vi "DigitalDemultiplexerV3.vi"() -> ()   [LabVIEW 2012]
uses:
  <vilib>/Platform/TimedLoop/XDataNode/timing_clust.ctl
  <vilib>/Platform/TimedLoop/XDataNode/nitl_modes.ctl
  <vilib>/Platform/TimedLoop/XDataNode/wakeup.ctl
  <vilib>/rvi/Emulation/niFpgaSctlEmulationRegisterWithScheduler.vi
  <vilib>/rvi/eio/common/nirviEmuTemplateMethod_errors.vi
  <vilib>/rvi/Emulation/niFpgaSctlEmulationScheduler.vi
  <vilib>/rvi/FIFO/Fifo_Resource/nirvififoEmulationSetSize.vi
  <vilib>/rvi/DataTransferAndStorage/Container/Common/niFpgaContainerGetUniqueNameForEmu.vi
  <vilib>/rvi/errors/niFpgaSetErrorForExecOnDevCompSimple.vi
  <vilib>/rvi/eio/common/nirviEmuReportErrorAndStop.vi
  <vilib>/rvi/Emulation/niFpgaSctlEmulationFifoFullMgr.vi
  <vilib>/rvi/Emulation/niFpgaSctlEmulationResourceMgr.vi
  <vilib>/rvi/interface/RandomDataEmulation/nirviRandomDataFPGAFIFO.vi
  <vilib>/rvi/interface/RandomDataEmulation/niFpgaRandomDataHandleErrors.vi
  <vilib>/rvi/Emulation/niFpgaSctlEmulationGlobalWrite.vi
  <vilib>/Platform/TimedLoop/XDataNode/XDataNode.xnode
  <vilib>/eio/EIONode/EIONode.xnode
  <vilib>/rvi/DataTransferAndStorage/Container/XNode/niFpgaContainer.xnode
  <vilib>/rvi/FIFO/Fifo_Resource/nirvififoEmulationClear.vi
  <vilib>/rvi/FIFO/Fifo_Resource/nirvififoEmulationWrite.vi
  <vilib>/rvi/FIFO/Fifo_Resource/nirvififoEmulationRead.vi
  <vilib>/rvi/interface/RandomDataEmulation/nirviRandomDataFpgaReadWriteTemplate.vi
  <vilib>/Platform/TimedLoop/XDataNode/XDNodeRunTimeDep.lvlib
panel:
  in  "Count mode":bool
  out "Laser pulses per pixel A1":u16
  out "ToHost FIFO Overflow A2Ch2":bool
  out "ToHost FIFO Overflow A2Ch1":bool
  out "ToHost FIFO Overflow A1Ch2":bool
  in  "Samples per pixel Acq A2":u16=10000 caption="Samples per pixel Acq"
  in  "Samples per pixel Acq A1":u16=10000 caption="Samples per pixel Acq"
  in  "Requested pixels A2":u32=100000 caption="Requested pixels"
  in  "Samples per pixel A2":u16=10000 caption="Samples per pixel"
  out "ToHost FIFO Overflow A1Ch1":bool
  out "Acquiring":bool
  in  "Wait for trigger":bool
  in  "Acquire continuously":bool=TRUE
  in  "Requested pixels A1":u32=100000 caption="Requested pixels"
  in  "Clear Interloop FIFO":bool
  out "Interloop FIFO overflow":bool
  in  "Samples per pixel A1":u16=10000 caption="Samples per pixel"
  in  "Acquire":bool
  out "Interloop FIFO timeout":bool
  in  "Commit":bool
  out "Xpoint_Switch_Ready":bool
  in  "Xpoint_Switch_Write":bool
  in  "Clock Source":u8(ring)=3 items=["Tristate"=0, "Sync Clock (PXIe only)"=2, "Adapter Module Onboard Clock"=3, "Strobe from Crosspoint Switch"=4, "Strobe Bypass"=5]
  in  "Onboard_Clock_Write":bool
  in  "Onboard_Clock_Write_Data":u16
  out "Onboard_Clock_Ready":bool
  in  "Acq_Reset":bool
  # "6587 IO module configuration"
  # "Digital Demultiplexer V3 - very simple 160, count high or flanks"
  # "Acquisition control"
  # "Area 1"
  # "Area 2"
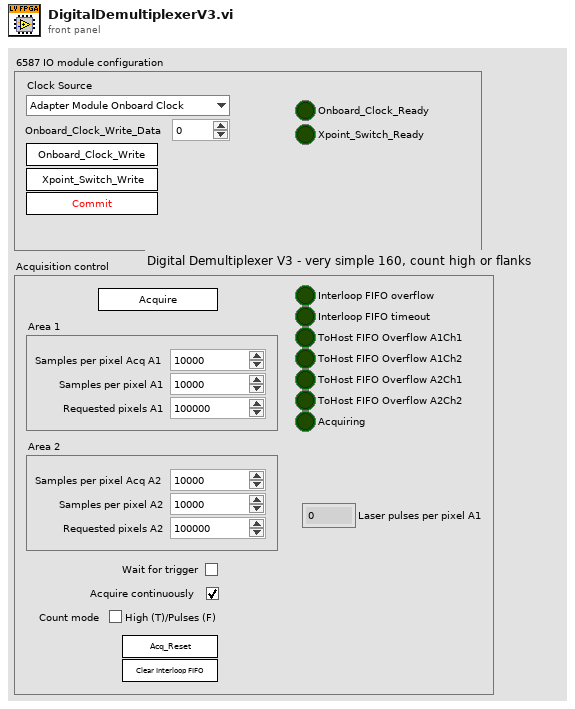
[diagram p1: front panel]
types:
  T1 = typedef "XDNodeRunTimeDep.lvlib/timing_clust.ctl" = cluster{"Expected End [f-1]":u64, "Actual End [f-1]":u64, "Finished Late? [f-1]":bool, "Expected End [i-1]":u64, "Actual End [i-1]":u64, "Finished Late? [i-1]":bool, "Expected Start [i]":u64, "Actual Start [i]":u64, "Expected Start [f]":u64, "Actual Start [f]":u64, "Source Name":string, "Structure Name":string, "Period":i64, "Deadline":i64, "Offset":i64, "Start":i64, "Priority":i32, "Timeout":i32, "Mode":T2, "Wakeup Reason":T3, "Error":errorcluster, "Source Type":string, "Secondary Source Type":string, "Global End Time":u64, "Global Start Time":u64, "Frame Duration":u64, "Iteration Duration":u64, "Assigned CPU":i32, "I/O Scan Engine Mode":u32}
  T2 = typedef "XDNodeRunTimeDep.lvlib/nitl_modes.ctl" = enum32{"No Change", "Process missed periods, maintain original phase", "Discard missed periods, maintain original phase", "Process missed periods, ignore original phase", "Discard missed periods, ignore original phase"}
  T3 = typedef "XDNodeRunTimeDep.lvlib/wakeup.ctl" = enum32{"Normal", "Aborted", "Asynchronous wakeup", "Timing source error", "Timed loop error", "Timeout"}
  T4 = cluster{"Laser":u64, "A1Ch1":u64, "A1Ch2":u64, "A2Ch1":u64, "A2Ch2":u64}
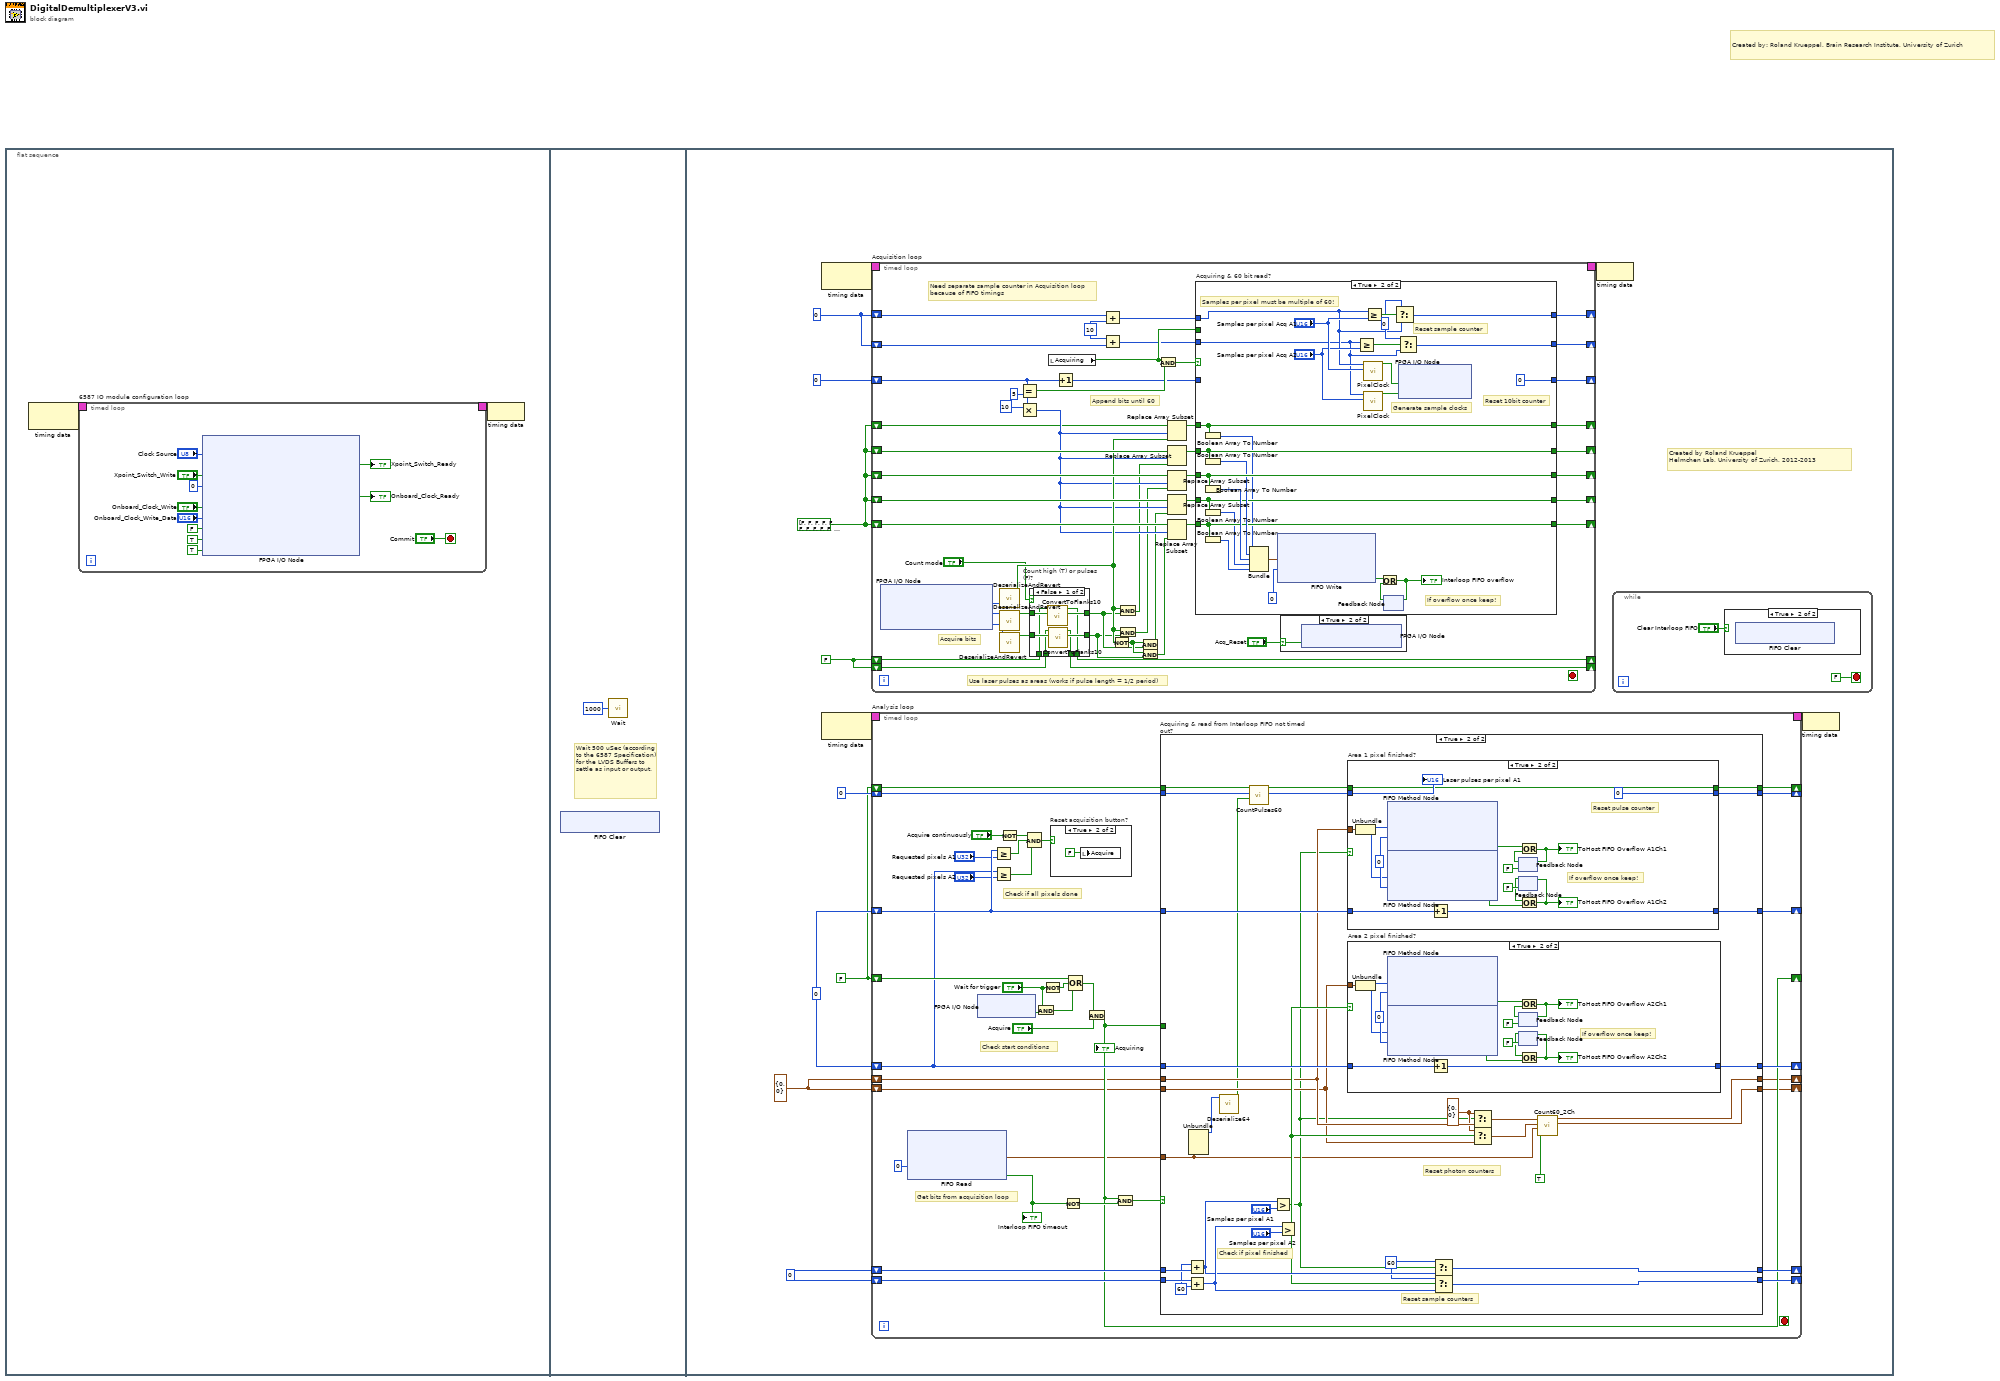
[diagram p0: block diagram]
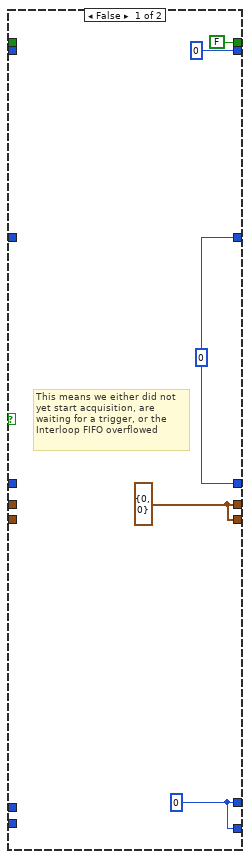
[diagram p5: hidden frame]
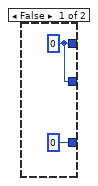
[diagram p11: hidden frame]
diagram:
  # "Created by: Roland Krueppel, Brain Research Institute, University of Zurich"
  n1 = flat-sequence {
    frame #0 {
      n2 = node-c288() -> (w2:T1)  [unwired: 1 in]
      n3 = timed-loop "6587 IO module configuration loop" {
        timing: w2 -> [_]
        timing-out: [_] -> w1
        stop <- "Commit" stop-if-true
        n4 = xnode "FPGA I/O Node"("IO Module\\Acq_IO_Clock_Source"="Clock Source", "IO Module\\Xpoint_Switch_Write"="Xpoint_Switch_Write", "IO Module\\LVDS_Data_Dir"=u16 0 ("IO Module\\LVDS_Data_Dir"), "IO Module\\Onboard_Clock_Write"="Onboard_Clock_Write", "IO Module\\Onboard_Clock_Write_Data"="Onboard_Clock_Write_Data", "IO Module\\SE_PFI0_WE"=FALSE ("IO Module\\SE_PFI0_WE"), "IO Module\\SE_PFI1_WE"=TRUE ("IO Module\\SE_PFI1_WE"), "IO Module\\SE_PFI2_WE"=TRUE ("IO Module\\SE_PFI2_WE")) -> ("IO Module\\Xpoint_Switch_Ready"=→"Xpoint_Switch_Ready":bool, "IO Module\\Onboard_Clock_Ready"=→"Onboard_Clock_Ready":bool)  [unwired: 10 in, 10 out]
      }
      n5 = node-c288(w1) -> ()
    }
    frame #1 {
      # "Wait 500 uSec (according to the 6587 Specification) for the LVDS Buffers to settle as input or output."
      n6 = xnode ("FIFO Clear")() -> ()  [unwired: 1 in, 1 out]
      n7 = call "Wait"("Count(uSec)"=u32 1000) -> ()  [unwired: 1 out]
    }
    frame #2 {
      w19 = FALSE
      w24 = cluster{u16, u16} {0, 0} ("output cluster")
      w25 = u16 0
      w23 = u32 0 ("Cycle counter out")
      w26 = u16 0
      w22 = bool[] [FALSE, FALSE, FALSE, FALSE, FALSE, FALSE, FALSE, FALSE, FALSE, FALSE, FALSE, FALSE, FALSE, FALSE, FALSE, FALSE, FALSE, FALSE, FALSE, FALSE, FALSE, FALSE, FALSE, FALSE, FALSE, FALSE, FALSE, FALSE, FALSE, FALSE, FALSE, FALSE, FALSE, FALSE, FALSE, FALSE, FALSE, FALSE, FALSE, FALSE, FALSE, FALSE, FALSE, FALSE, FALSE, FALSE, FALSE, FALSE, FALSE, FALSE, FALSE, FALSE, FALSE, FALSE, FALSE, FALSE, FALSE, FALSE, FALSE, FALSE, FALSE, FALSE, FALSE, FALSE] ("Boolean array")
      w20 = FALSE ("Last laser bit out")
      # "Created by Roland Krueppel\nHelmchen Lab, University of Zurich, 2012-2013"
      n8 = node-c288() -> (w31:T1)  [unwired: 1 in]
      n9 = node-c288() -> (w29:T1)  [unwired: 1 in]
      n10 = timed-loop "Acquisition loop" {
        timing: w31 -> [_]
        timing-out: [_] -> w30
        shift-right: [w216] -> _
        shift-left: w22 -> [w222]
        shift-right: [w215] -> _
        shift-left: 0 -> [w214]
        shift-right: [w211] -> _
        shift-left: w22 -> [w213]
        shift-right: [w210] -> _
        shift-left: w25 -> [w203]
        shift-right: [w209] -> _
        shift-left: w25 -> [w201]
        shift-right: [w192] -> _
        shift-left: w22 -> [w197]
        shift-right: [w191] -> _
        shift-left: w22 -> [w196]
        shift-right: [w186] -> _
        shift-left: w22 -> [w188]
        shift-right: [w175] -> _
        shift-left: w19 -> [w177]
        shift-right: [w174] -> _
        shift-left: w19 -> [w176]
        stop <- _ stop-if-true
        w199 = u16 10 ("y")
        # "Use laser pulses as areas (works if pulse length = 1/2 period)"
        # "Need separate sample counter in Acquisition loop\nbecause of FIFO timings"
        # "Append bits until 60"
        # "Acquire bits"
        n11 = xnode "FPGA I/O Node"() -> ("IO Module\\LVDS_Ch0_Rd"=w206:u16, "IO Module\\LVDS_Ch1_Rd"=w205:u16, "IO Module\\LVDS_Ch2_Rd"=w204:u16)  [unwired: 3 in, 3 out]
        n12 = call "DeserializeAndRevert.vi"("U16 input"=w206) -> ("10bit output"=w190:bool[])  [unwired: 10 in]
        n13 = call "DeserializeAndRevert.vi"("U16 input"=w205) -> ("10bit output"=w181:bool[])  [unwired: 10 in]
        n14 = call "DeserializeAndRevert.vi"("U16 input"=w204) -> ("10bit output"=w180:bool[])  [unwired: 10 in]
        n15 = Equal?(x=w214, y=5) -> (x = y?=w219:bool)
        n16 = Multiply(x=10 ("y"), y=w214) -> (x*y=w189:i32)
        n17 = case "Count high (T) or pulses (F)?" shown="False" "Count mode" {
          tunnel: w181 -> [w230 w234]
          tunnel: w180 -> [w228 w233]
          tunnel: [w229 w234] -> w179
          tunnel: [w227 w233] -> w178
          tunnel: w177 -> [w226 w231]
          tunnel: w176 -> [w225 w232]
          tunnel: [w224 w232] -> w174
          tunnel: [w223 w231] -> w175
          frame False {
            n18 = call "ConvertToFlanks10.vi"("10bit input"=w230, "Last sample in"=w226) -> ("Flank output"=w229:bool[], "Last sample out"=w223:bool)  [unwired: 8 in]
            n19 = call "ConvertToFlanks10.vi"("10bit input"=w228, "Last sample in"=w225) -> ("Flank output"=w227:bool[], "Last sample out"=w224:bool)  [unwired: 8 in]
          }
          frame True {
          }
        }
        n20 = local read "Acquiring"() -> (w208:bool)
        n21 = Increment(x=w214) -> (x+1=w207:i32)
        n22 = Add(x=w203, y=w199) -> (x+y=w202:u16)
        n23 = Add(x=w199, y=w201) -> (x+y=w200:u16)
        n24 = Not(x=w190) -> (.not. x?=w195:bool[])
        n25 = And(x=w190, y=w179) -> (x .and. y?=w185:bool[])
        n26 = And(x=w190, y=w178) -> (x .and. y?=w184:bool[])
        n27 = And(x=w195, y=w179) -> (x .and. y?=w183:bool[])
        n28 = And(x=w195, y=w178) -> (x .and. y?=w182:bool[])
        n29 = And(x=w208, y=w219) -> (x .and. y?=w218:bool)
        n30 = Replace Array Subset(array=w188, new element=w190, index=w189) -> (w187:bool[])
        n31 = Replace Array Subset(array=w222, new element=w185, index=w189) -> (w217:bool[])
        n32 = Replace Array Subset(array=w213, new element=w184, index=w189) -> (w212:bool[])
        n33 = Replace Array Subset(array=w197, new element=w183, index=w189) -> (w194:bool[])
        n34 = Replace Array Subset(array=w196, new element=w182, index=w189) -> (w193:bool[])
        n35 = case "Acquiring & 60 bit read?" shown="True" w218 {
          tunnel: w217 -> [w247 w278]
          tunnel: [w247 w278] -> w216
          tunnel: [w239 0] -> w215
          tunnel: w207 -> [w240 _]
          tunnel: w212 -> [w246 w277]
          tunnel: [w246 w277] -> w211
          tunnel: w202 -> [w244 w266]
          tunnel: [w241 w275] -> w210
          tunnel: w200 -> [w243 w265]
          tunnel: [w242 w270] -> w209
          tunnel: w208 -> [w245 _]
          tunnel: w194 -> [w238 w259]
          tunnel: w193 -> [w237 w258]
          tunnel: [w238 w259] -> w192
          tunnel: [w237 w258] -> w191
          tunnel: w187 -> [w236 w254]
          tunnel: [w236 w254] -> w186
          frame False {
            n36 = case "Acquiring?" shown="True" w245 {
              tunnel: w244 -> [_ w252]
              tunnel: w243 -> [_ w251]
              tunnel: [w249 w252] -> w241
              tunnel: [w249 w251] -> w242
              tunnel: w240 -> [_ w250]
              tunnel: [0 w250] -> w239
              frame False {
                w249 = u16 0
              }
              frame True {
              }
            }
          }
          frame True {
            w271 = u16 0 ("t")
            # "Reset 10bit counter"
            # "Samples per pixel must be multiple of 60!"
            # "Reset sample counter"
            # "If overflow once keep!"
            # "Generate sample clocks"
            n37 = Boolean Array To Number(Boolean array=w254) -> (number=w253:u64)
            n38 = Boolean Array To Number(Boolean array=w278) -> (number=w261:u64)
            n39 = Boolean Array To Number(Boolean array=w277) -> (number=w260:u64)
            n40 = Boolean Array To Number(Boolean array=w259) -> (number=w257:u64)
            n41 = Boolean Array To Number(Boolean array=w258) -> (number=w256:u64)
            n42 = Bundle(w253, w261, w260, w257, w256) -> (w255:cluster{u64, u64, u64, u64, u64})  [unwired: 1 in]
            n43 = xnode ("FIFO Write")("Element"=w255, "Timeout"=0) -> ("Timed Out?"=w264:bool)  [unwired: 1 in, 1 out]
            n44 = Greater Or Equal?(x=w265, y="Samples per pixel Acq A2") -> (x >= y?=w272:bool)
            n45 = call "PixelClock.vi"("Samples per pixel"="Samples per pixel Acq A1", "Sample counter"=w266) -> ("Pixel clock"=w273:bool)  [unwired: 9 in]
            n46 = call "PixelClock.vi"("Samples per pixel"="Samples per pixel Acq A2", "Sample counter"=w265) -> ("Pixel clock"=w268:bool)  [unwired: 9 in]
            n47 = Greater Or Equal?(x=w266, y="Samples per pixel Acq A1") -> (x >= y?=w276:bool)
            n48 = feedback #1() -> (w262:bool)  [unwired: 1 in]
            n49 = Or(x=w264, y=w262) -> (x .or. y?=w263:bool)
            "Interloop FIFO overflow" <- w263
            n50 = feedback-in #1(w263) -> ()
            n51 = Select(t=w271, s=w276, f=w266) -> (s? t:f=w275:u16)
            n52 = Select(t=w271, s=w272, f=w265) -> (s? t:f=w270:u16)
            n53 = xnode "FPGA I/O Node"("Pixel clock A1"=w273, "Pixel clock A2"=w268) -> ()  [unwired: 2 in, 2 out]
          }
        }
        n54 = case shown="True" "Acq_Reset" {
          selector: "Acq_Reset" -> [_ w235]
          frame False {
          }
          frame True {
            n55 = xnode "FPGA I/O Node"("IO Module\\Acq_Reset"=w235) -> ()  [unwired: 1 in, 1 out]
          }
        }
      }
      n56 = timed-loop "Analysis loop" {
        timing: w29 -> [_]
        timing-out: [_] -> w28
        shift-right: [w49] -> _
        shift-left: w26 -> [w69]
        shift-right: [w47] -> _
        shift-left: w23 -> [w68]
        shift-right: [w45] -> _
        shift-left: w20 -> [w57]
        shift-right: [w48] -> _
        shift-left: w26 -> [w55]
        shift-right: [w46] -> _
        shift-left: w23 -> [w53]
        shift-right: [w40] -> _
        shift-left: w24 -> [w42]
        shift-right: [w39] -> _
        shift-left: w24 -> [w41]
        shift-right: [w37] -> _
        shift-left: u16 0 ("New pulse count") -> [w36]
        shift-right: [w35] -> _
        shift-left: w20 -> [w34]
        stop <- _ stop-if-true
        # "Get bits from acquisition loop"
        # "Check start conditions"
        # "Check if all pixels done"
        n57 = xnode ("FIFO Read")("Timeout"=0) -> ("Element"=w38:T4, "Timed Out?"=w43:bool)  [unwired: 1 in, 1 out]
        "Interloop FIFO timeout" <- w43
        n58 = xnode "FPGA I/O Node"() -> ("TriggerIn"=w63:bool)  [unwired: 1 in, 1 out]
        n59 = Greater Or Equal?(x=w68, y="Requested pixels A1") -> (x >= y?=w51:bool)
        n60 = Greater Or Equal?(x=w53, y="Requested pixels A2") -> (x >= y?=w50:bool)
        n61 = Not(x="Acquire continuously") -> (.not. x?=w52:bool)
        n62 = Compound Arithmetic op=AND(w52, w51, w50) -> (w65:bool)
        n63 = And(x="Wait for trigger", y=w63) -> (x .and. y?=w60:bool)
        n64 = Not(x="Wait for trigger") -> (.not. x?=w61:bool)
        n65 = case "Reset acquisition button?" shown="True" w65 {
          frame False {
          }
          frame True {
            n66 = local write "Acquire"(FALSE ("Acquire")) -> ()
          }
        }
        n67 = Not(x=w43) -> (.not. x?=w58:bool)
        n68 = Compound Arithmetic op=OR(w57, w61, w60) -> (w59:bool)
        n69 = And(x=w59, y="Acquire") -> (x .and. y?=w45:bool)
        "Acquiring" <- w45
        n70 = And(x=w45, y=w58) -> (x .and. y?=w56:bool)
        n71 = case "Acquiring & read from Interloop FIFO not timed out?" shown="True" w56 {
          tunnel: w42 -> [w86 w118]
          tunnel: w69 -> [w85 w133]
          tunnel: w68 -> [w84 w129]
          tunnel: w45 -> [w87 _]
          tunnel: w55 -> [w78 w131]
          tunnel: w53 -> [w81 w128]
          tunnel: [w79 w121] -> w49
          tunnel: [w77 w123] -> w48
          tunnel: [w83 w112] -> w40
          tunnel: [w82 w126] -> w47
          tunnel: [w80 w127] -> w46
          tunnel: w41 -> [w76 w117]
          tunnel: [w75 w111] -> w39
          tunnel: w38 -> [_ w110]
          tunnel: [w71 w105] -> w37
          tunnel: w36 -> [w73 w104]
          tunnel: [w72 w103] -> w35
          tunnel: w34 -> [w74 w102]
          frame False {
            n72 = case "Acquiring?" shown="True" w87 {
              tunnel: w86 -> [_ w100]
              tunnel: w85 -> [_ w97]
              tunnel: w84 -> [_ w99]
              tunnel: [w91 w100] -> w83
              tunnel: [w92 w99] -> w82
              tunnel: w81 -> [_ w98]
              tunnel: [w92 w98] -> w80
              tunnel: [w90 w97] -> w79
              tunnel: [w90 w96] -> w77
              tunnel: w78 -> [_ w96]
              tunnel: w76 -> [_ w95]
              tunnel: [w91 w95] -> w75
              tunnel: w74 -> [_ w94]
              tunnel: w73 -> [_ w93]
              tunnel: [FALSE ("Last laser bit out") w94] -> w72
              tunnel: [u16 0 ("New pulse count") w93] -> w71
              frame False {
                w91 = cluster{u16, u16} {0, 0} ("output cluster")
                w92 = u32 0 ("Cycle counter out")
                w90 = u16 0
                # "This means we either did not\nyet start acquisition, are\nwaiting for a trigger, or the\nInterloop FIFO overflowed"
              }
              frame True {
                # "This means we are\nreading faster here\nthan acquiring in\nAcquisition loop\n-> keep all values"
              }
            }
          }
          frame True {
            w116 = cluster{u16, u16} {0, 0} ("t")
            w120 = u16 60 ("t")
            w130 = u16 60
            # "Reset photon counters"
            # "Check if pixel finished"
            # "Reset sample counters"
            n73 = Add(x=w130, y=w133) -> (x+y=w122:u16)
            n74 = Add(x=w131, y=w130) -> (x+y=w124:u16)
            n75 = Unbundle(w110) -> ("Laser"=w109:u64)  [unwired: 4 out]
            n76 = call "Deserialize64.vi"("U64 input"=w109) -> ("60bit output"=w108:bool[])  [unwired: 10 in]
            n77 = call "CountPulses60.vi"("60bit input"=w108, "Previous pulse count"=w104, "Last sample"=w102) -> ("New pulse count"=w107:u16, "New last sample"=w106:bool)  [unwired: 7 in]
            n78 = Greater?(x=w122, y="Samples per pixel A1") -> (0:w115:bool)
            n79 = Greater?(x=w124, y="Samples per pixel A2") -> (0:w119:bool)
            n80 = case "Area 1 pixel finished?" shown="True" w115 {
              tunnel: w118 -> [_ w165]
              tunnel: w129 -> [w151 w167]
              tunnel: [w151 w166] -> w126
              tunnel: w107 -> [w149 w154]
              tunnel: w106 -> [w150 w153]
              tunnel: [w149 u16 0 ("New pulse count")] -> w105
              tunnel: [w150 w153] -> w103
              frame False {
              }
              frame True {
                w168 = 0 ("Timeout")
                # "Reset pulse counter"
                # "If overflow once keep!"
                n81 = Unbundle(w165) -> (w164:u16, w163:u16)
                n82 = xnode ("FIFO Method Node")("Element"=w164, "Timeout"=w168) -> ("Timed Out?"=w158:bool)  [unwired: 1 in, 1 out]
                n83 = xnode ("FIFO Method Node")("Element"=w163, "Timeout"=w168) -> ("Timed Out?"=w157:bool)  [unwired: 1 in, 1 out]
                n84 = Increment(x=w167) -> (x+1=w166:u32)
                n85 = feedback #2(FALSE) -> (w162:bool)
                n86 = feedback #3(FALSE) -> (w159:bool)
                n87 = Or(x=w158, y=w162) -> (x .or. y?=w156:bool)
                "ToHost FIFO Overflow A1Ch1" <- w156
                n88 = feedback-in #2(w156) -> ()
                n89 = Or(x=w159, y=w157) -> (x .or. y?=w155:bool)
                "ToHost FIFO Overflow A1Ch2" <- w155
                n90 = feedback-in #3(w155) -> ()
                "Laser pulses per pixel A1" <- w154
              }
            }
            n91 = case "Area 2 pixel finished?" shown="True" w119 {
              tunnel: w128 -> [w134 w147]
              tunnel: [w134 w146] -> w127
              tunnel: w117 -> [_ w145]
              frame False {
              }
              frame True {
                w148 = 0 ("Timeout")
                # "If overflow once keep!"
                n92 = Unbundle(w145) -> (w144:u16, w143:u16)
                n93 = xnode ("FIFO Method Node")("Element"=w144, "Timeout"=w148) -> ("Timed Out?"=w138:bool)  [unwired: 1 in, 1 out]
                n94 = xnode ("FIFO Method Node")("Element"=w143, "Timeout"=w148) -> ("Timed Out?"=w137:bool)  [unwired: 1 in, 1 out]
                n95 = Increment(x=w147) -> (x+1=w146:u32)
                n96 = feedback #4(FALSE) -> (w142:bool)
                n97 = feedback #5(FALSE) -> (w139:bool)
                n98 = Or(x=w138, y=w142) -> (x .or. y?=w136:bool)
                "ToHost FIFO Overflow A2Ch1" <- w136
                n99 = feedback-in #4(w136) -> ()
                n100 = Or(x=w139, y=w137) -> (x .or. y?=w135:bool)
                "ToHost FIFO Overflow A2Ch2" <- w135
                n101 = feedback-in #5(w135) -> ()
              }
            }
            n102 = Select(t=w120, s=w115, f=w122) -> (s? t:f=w121:u16)
            n103 = Select(t=w120, s=w119, f=w124) -> (s? t:f=w123:u16)
            n104 = Select(t=w116, s=w115, f=w118) -> (s? t:f=w114:cluster{u16, u16})
            n105 = Select(t=w116, s=w119, f=w117) -> (s? t:f=w113:cluster{u16, u16})
            n106 = call "Count60_2Ch.vi"("Count type"=TRUE, "Area interloop cluster"=w110, "Photon counters area 2 in"=w113, "Photon counters area 1 in"=w114) -> ("Photon counters area 2 out"=w111:cluster{u16, u16}, "Photon counters area 1 out"=w112:cluster{u16, u16})  [unwired: 5 in, 1 out]
          }
        }
      }
      n107 = node-c288(w30) -> ()
      n108 = while {
        stop <- FALSE stop-if-true
        n109 = case shown="True" "Clear Interloop FIFO" {
          frame False {
          }
          frame True {
            n110 = xnode ("FIFO Clear")() -> ()  [unwired: 1 in, 1 out]
          }
        }
      }
      n111 = node-c288(w28) -> ()
    }
  }
